vi "string-unbundler.vi"(0 "String":string) -> (1 "Array 1":dbl[](array[numeric]), 2 "Array 2":dbl[](array[numeric]))   [LabVIEW 2023]
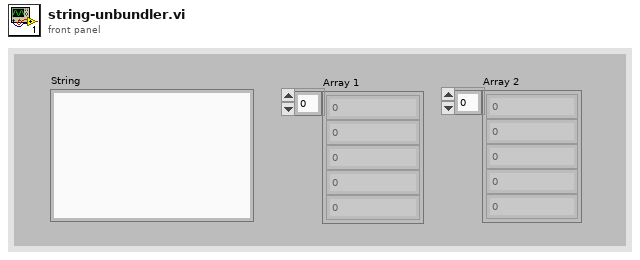
[diagram p1: front panel]
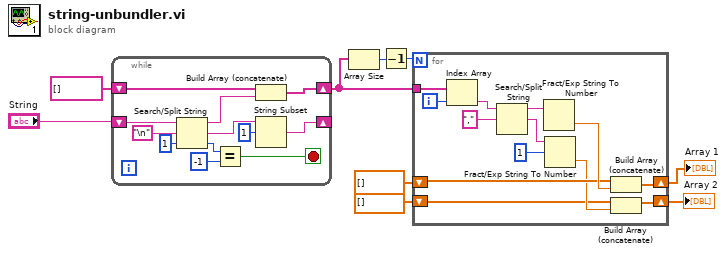
[diagram p0: block diagram]
diagram:
  n1 = while {
    shift-right: [w18] -> w9
    shift-left: string[] [] -> [w20]
    shift-right: [w12] -> _
    shift-left: "String" -> [w19]
    stop <- w15 stop-if-true
    n2 = Search/Split String(string=w19, search string/char (-)="\n", offset (0)=1) -> (substring before match=w21:string, match + rest of string=w13:string, offset of match=w17:i32)
    n3 = Equal?(x=w17, y=-1) -> (x = y?=w15:bool)
    n4 = Build Array (concatenate)(w20, w21) -> (w18:string[])
    n5 = String Subset(string=w13, offset (0)=1) -> (substring=w12:string)  [unwired: 1 in]
  }
  n6 = Array Size(array=w9) -> (size(s)=w1:i32)
  n7 = Decrement(x=w1) -> (x-1=w2:i32)
  n8 = for {
    N: w2 -> [_]
    tunnel: w9 -> [w34]
    shift-right: [w23] -> w6
    shift-left: dbl[] [] -> [w26]
    shift-right: [w28] -> w5
    shift-left: dbl[] [] -> [w24]
    i -> [w33]
    n9 = Index Array(array=w34, index=w33) -> (element=w32:string)
    n10 = Search/Split String(string=w32, search string/char (-)=",") -> (substring before match=w30:string, match + rest of string=w29:string)  [unwired: 1 in, 1 out]
    n11 = Fract/Exp String To Number(string=w30) -> (number=w27:dbl)  [unwired: 3 in, 1 out]
    n12 = Fract/Exp String To Number(string=w29, offset=1) -> (number=w25:dbl)  [unwired: 2 in, 1 out]
    n13 = Build Array (concatenate)(w26, w27) -> (w23:dbl[])
    n14 = Build Array (concatenate)(w24, w25) -> (w28:dbl[])
  }
  "Array 1" <- w6
  "Array 2" <- w5
